vi "Expand the Compact PDO.vi"(8 "error in (no error)":errorcluster, 10 "Arr Refnum":refnum<vi>, 11 "File Refnum":T1) -> (0 "error out":errorcluster, 2 "dup File Refnum":T1, 3 "dup Arr Refnum":refnum<vi>)   [LabVIEW 2013]
uses:
  <vilib>/Utility/config.llb/Config Data RefNum.ctl
  <vilib>/Utility/config.llb/Read Key (String).vi
  <vilib>/Utility/config.llb/NI_LVConfig.lvlib
panel:
  in  "CompactPDO":u8 format="%.0x"
  in  "NrOfTXPDO":u16
  in  "NrOfRXPDO":u16
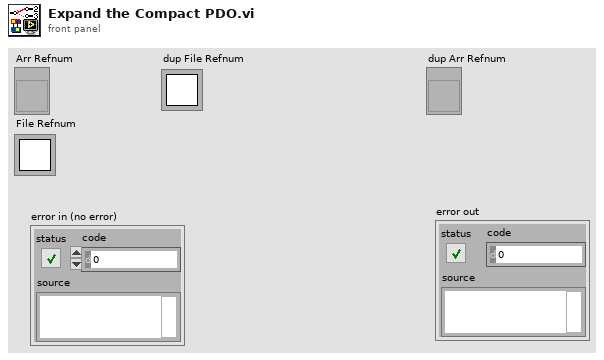
[diagram p1: front panel]
types:
  T1 = typedef "NI_LVConfig.lvlib/Config Data RefNum.ctl" = refnum<k1>
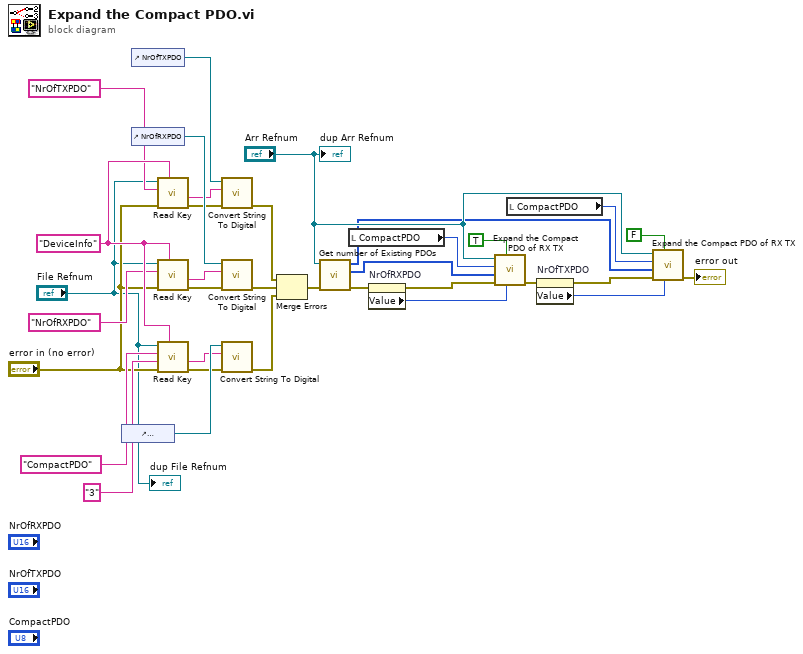
[diagram p0: block diagram]
diagram:
  w32 = "DeviceInfo" ("section")
  n1 = control-ref of="CompactPDO"() -> (w29:refnum<vi>)
  n2 = control-ref of="NrOfTXPDO"() -> (w23:refnum<vi>)
  n3 = control-ref of="NrOfRXPDO"() -> (w25:refnum<vi>)
  n4 = call-poly <vilib>:"Read Key.vi"("section"=w32, "error in (no error)"="error in (no error)", "key"="NrOfTXPDO", "refnum"="File Refnum") -> ("error out"=w21:errorcluster, "value"=w22:string)  [unwired: 4 in, 2 out]
  n5 = call-poly <vilib>:"Read Key.vi"("section"=w32, "error in (no error)"="error in (no error)", "key"="NrOfRXPDO", "refnum"="File Refnum") -> ("error out"=w26:errorcluster, "value"=w24:string)  [unwired: 4 in, 2 out]
  n6 = call-poly <vilib>:"Read Key.vi"("section"=w32, "error in (no error)"="error in (no error)", "default value"="3", "key"="CompactPDO", "refnum"="File Refnum") -> ("error out"=w27:errorcluster, "value"=w28:string)  [unwired: 3 in, 2 out]
  n7 = call "Convert String To Digital.vi"("error in (no error)"=w21, "Value"=w22, "DigNum Refnum"=w23) -> ("error out"=w18:errorcluster)  [unwired: 8 in]
  n8 = call "Convert String To Digital.vi"("error in (no error)"=w26, "Value"=w24, "DigNum Refnum"=w25) -> ("error out"=w19:errorcluster)  [unwired: 8 in]
  n9 = call "Convert String To Digital.vi"("error in (no error)"=w27, "Value"=w28, "DigNum Refnum"=w29) -> ("error out"=w17:errorcluster)  [unwired: 8 in]
  n10 = Merge Errors(w18, w19, w17) -> (w14:errorcluster)
  n11 = call "Get number of Existing PDOs.vi"("error in (no error)"=w14, "Arr Refnum"="Arr Refnum") -> ("error out"=w13:errorcluster, "RX PDOs"=w1:u16[], "TX PDOs"=w2:u16[])  [unwired: 7 in]
  n12 = local read "CompactPDO"() -> (w8:u8)
  n13 = property on="NrOfRXPDO" class="DigNum (strict)"(error in=w13) -> (error out=w11:errorcluster, "Value"=w3:u16)  [unwired: 1 in, 1 out]
  n14 = call "Expand the Compact PDO of RX TX.vi"("Number"=w3, "RX?"=TRUE, "error in (no error)"=w11, "Existing Indexs"=w1, "CompactPDO"=w8, "Arr Refnum"="Arr Refnum") -> ("error out"=w10:errorcluster)  [unwired: 5 in]
  n15 = local read "CompactPDO"() -> (w6:u8)
  n16 = property on="NrOfTXPDO" class="DigNum (strict)"(error in=w10) -> (error out=w9:errorcluster, "Value"=w4:u16)  [unwired: 1 in, 1 out]
  n17 = call "Expand the Compact PDO of RX TX.vi"("Number"=w4, "RX?"=FALSE, "error in (no error)"=w9, "Existing Indexs"=w2, "CompactPDO"=w6, "Arr Refnum"="Arr Refnum") -> ("error out"=→"error out":errorcluster)  [unwired: 5 in]
  "dup Arr Refnum" <- "Arr Refnum"
  "dup File Refnum" <- "File Refnum"
